vi "Post-Build Action.vi"(5 "Files Generated by Build":path[](array[path]), 6 "Top Level/Always Included VIs":path[](array[path]), 7 "Destination Path":path, 8 "error in (no error)":errorcluster, 9 "Target Name":string, 10 "Build Specification Name":string, 11 "Project Path":path) -> (0 "error out":errorcluster)   [LabVIEW 2018]
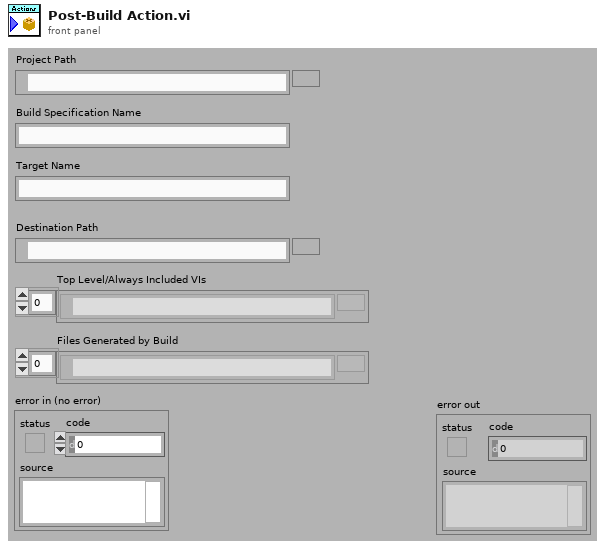
[diagram p1: front panel]
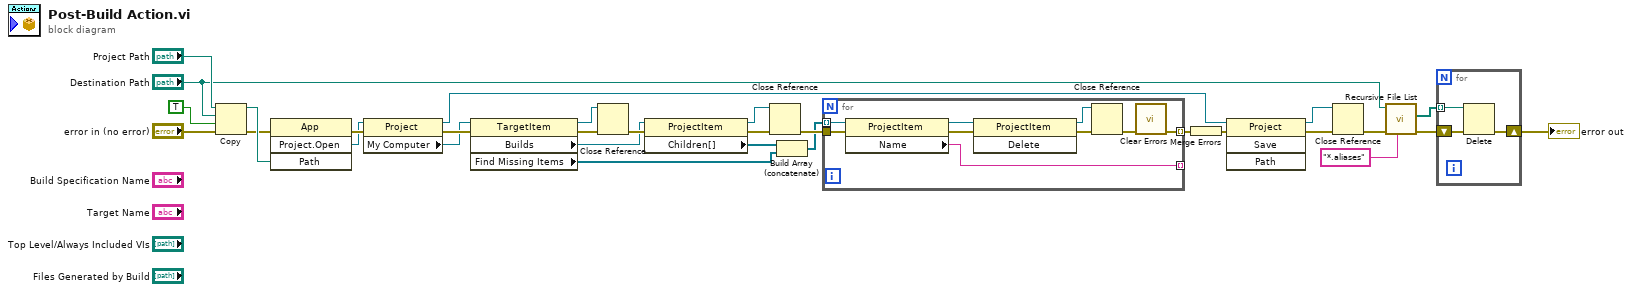
[diagram p0: block diagram]
diagram:
  n1 = Copy(8:"error in (no error)", 9:TRUE ("overwrite (F)"), 10:"Destination Path", 11:"Project Path") -> (0:w22:errorcluster, 3:w26:path)  [unwired: 1 in, 1 out]
  n2 = invoke class="App" method="Project.Open"(error in=w22, "Path"=w26) -> (error out=w23:errorcluster, "Project:Open"=w19:refnum<vi>)  [unwired: 2 in, 2 out]
  n3 = property class="Project"(reference=w19, error in=w23) -> (reference out=w25:refnum<vi>, error out=w24:errorcluster, "My Computer"=w18:refnum<vi>)
  n4 = property class="TargetItem"(reference=w18, error in=w24) -> (reference out=w6:refnum<vi>, error out=w7:errorcluster, "Builds"=w4:refnum<vi>, "Find Missing Items"=w2:refnum<vi>[])
  n5 = Close Reference(reference=w6, error in (no error)=w7) -> (error out=w5:errorcluster)
  n6 = property class="ProjectItem"(reference=w4, error in=w5) -> (reference out=w9:refnum<vi>, error out=w10:errorcluster, "Children[]"=w3:refnum<vi>[])
  n7 = Close Reference(reference=w9, error in (no error)=w10) -> (error out=w8:errorcluster)
  n8 = Build Array (concatenate)(w3, w2) -> (w1:refnum<vi>[])
  n9 = for {
    tunnel: w1 -> [w35] mode=indexing
    tunnel: [w33] -> _ mode=indexing
    tunnel: w8 -> [w37]
    tunnel: [w31] -> w11 mode=indexing
    n10 = property class="ProjectItem"(reference=w35, error in=w37) -> (reference out=w34:refnum<vi>, error out=w36:errorcluster, "Name"=w33:string)
    n11 = invoke class="ProjectItem" method="Delete"(reference=w34, error in=w36) -> (reference out=w38:refnum<vi>, error out=w39:errorcluster)  [unwired: 1 in, 1 out]
    n12 = Close Reference(reference=w38, error in (no error)=w39) -> (error out=w32:errorcluster)
    n13 = call <vilib>:"Clear Errors.vi"("error in (no error)"=w32) -> ("error out"=w31:errorcluster)  [unwired: 5 in, 1 out]
  }
  n14 = Merge Errors(w11) -> (w13:errorcluster)
  n15 = invoke class="Project" method="Save"(reference=w25, error in=w13) -> (reference out=w20:refnum<vi>, error out=w21:errorcluster)  [unwired: 2 in, 2 out]
  n16 = Close Reference(reference=w20, error in (no error)=w21) -> (error out=w17:errorcluster)
  n17 = call <vilib>:"Recursive File List.vi"("pattern"="*.aliases", "error in (no error)"=w17, "Folder Path"="Destination Path") -> ("error out"=w15:errorcluster, "All Files in Dir"=w14:path[])  [unwired: 4 in, 3 out]
  n18 = for {
    shift-right: [w40] -> w12
    shift-left: w15 -> [w42]
    tunnel: w14 -> [w41] mode=indexing
    n19 = Delete(path (use dialog)=w41, error in=w42) -> (error out=w40:errorcluster)  [unwired: 3 in, 2 out]
  }
  "error out" <- w12
